vi "Digital_Write_3_Lines_2011.vi"() -> ()   [LabVIEW 2011]
uses:
  <vilib>/DAQmx/write.llb/DAQmx Write (Digital Bool 1Line 1Point).vi
  <vilib>/DAQmx/create/channels.llb/DAQmx Create Channel (DO-Digital Output).vi
  <vilib>/DAQmx/miscellaneous.llb/DAQmx Fill In Error Info.vi
panel:
  in  "Stop":bool
  in  "Line 1 Data":bool
  in  "Line 2 Data":bool
  in  "Line 3 Data":bool
  in  "Output Line 3":tag="Dev1/port0/line2"
  in  "Output Line 2":tag="Dev1/port0/line1"
  in  "Output Line 1":tag="Dev1/port0/line0"
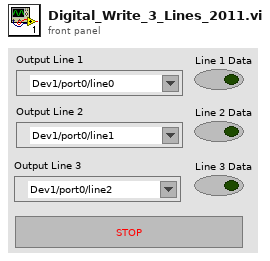
[diagram p1: front panel]
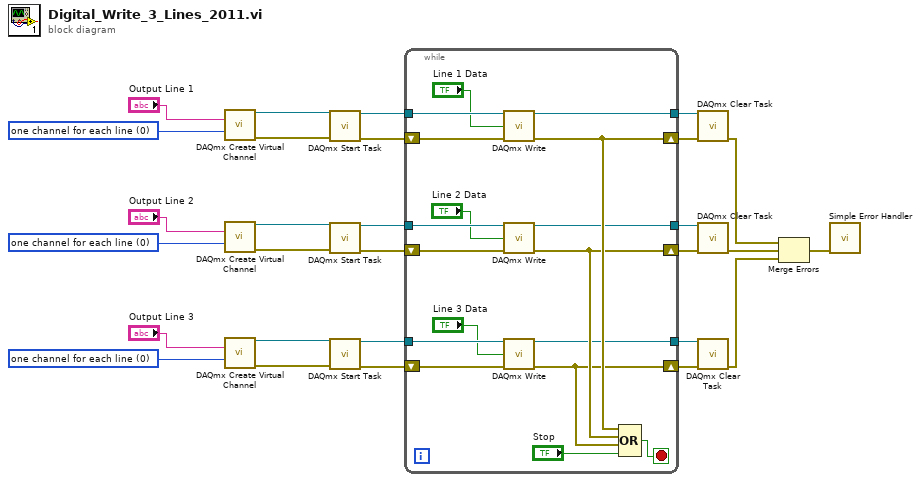
[diagram p0: block diagram]
diagram:
  w15 = 0 items=["one channel for each line", "one channel for all lines"] ("line grouping")
  w18 = 0 items=["one channel for each line", "one channel for all lines"] ("line grouping")
  w27 = 0 items=["one channel for each line", "one channel for all lines"] ("line grouping")
  n1 = call-poly <vilib>:"DAQmx Create Virtual Channel.vi"("lines"="Output Line 1", "line grouping"=w27) -> ("task out"=w26:refnum<k21>, "error out"=w25:errorcluster)  [unwired: 12 in]
  n2 = call-poly <vilib>:"DAQmx Create Virtual Channel.vi"("lines"="Output Line 2", "line grouping"=w18) -> ("task out"=w19:refnum<k21>, "error out"=w20:errorcluster)  [unwired: 12 in]
  n3 = call-poly <vilib>:"DAQmx Create Virtual Channel.vi"("lines"="Output Line 3", "line grouping"=w15) -> ("task out"=w14:refnum<k21>, "error out"=w13:errorcluster)  [unwired: 12 in]
  n4 = call <vilib>:"DAQmx Start Task.vi"("task/channels in"=w26, "error in"=w25) -> ("task out"=w24:refnum<k21>, "error out"=w23:errorcluster)  [unwired: 12 in]
  n5 = call <vilib>:"DAQmx Start Task.vi"("task/channels in"=w19, "error in"=w20) -> ("task out"=w21:refnum<k21>, "error out"=w22:errorcluster)  [unwired: 12 in]
  n6 = call <vilib>:"DAQmx Start Task.vi"("task/channels in"=w14, "error in"=w13) -> ("task out"=w12:refnum<k21>, "error out"=w11:errorcluster)  [unwired: 12 in]
  n7 = while {
    tunnel: w24 -> [w45]
    tunnel: w21 -> [w42]
    tunnel: w12 -> [w41]
    tunnel: [w31] -> w10
    tunnel: [w30] -> w8
    tunnel: [w29] -> w6
    shift-right: [w34] -> w7
    shift-left: w22 -> [w43]
    shift-right: [w35] -> w9
    shift-left: w23 -> [w44]
    shift-right: [w33] -> w5
    shift-left: w11 -> [w40]
    stop <- w36 stop-if-true
    n8 = call-poly <vilib>:"DAQmx Write.vi"("task/channels in"=w45, "data"="Line 1 Data", "error in"=w44) -> ("task out"=w31:refnum<k21>, "error out"=w35:errorcluster)  [unwired: 10 in, 1 out]
    n9 = call-poly <vilib>:"DAQmx Write.vi"("task/channels in"=w42, "data"="Line 2 Data", "error in"=w43) -> ("task out"=w30:refnum<k21>, "error out"=w34:errorcluster)  [unwired: 10 in, 1 out]
    n10 = call-poly <vilib>:"DAQmx Write.vi"("task/channels in"=w41, "data"="Line 3 Data", "error in"=w40) -> ("task out"=w29:refnum<k21>, "error out"=w33:errorcluster)  [unwired: 10 in, 1 out]
    n11 = Compound Arithmetic op=OR(w35, w34, w33, "Stop") -> (w36:bool)
  }
  n12 = call <vilib>:"DAQmx Clear Task.vi"("task in"=w10, "error in"=w9) -> ("error out"=w3:errorcluster)  [unwired: 13 in]
  n13 = call <vilib>:"DAQmx Clear Task.vi"("task in"=w8, "error in"=w7) -> ("error out"=w4:errorcluster)  [unwired: 13 in]
  n14 = call <vilib>:"DAQmx Clear Task.vi"("task in"=w6, "error in"=w5) -> ("error out"=w2:errorcluster)  [unwired: 13 in]
  n15 = Merge Errors(w3, w4, w2) -> (w1:errorcluster)
  n16 = call <vilib>:"Simple Error Handler.vi"("error in (no error)"=w1) -> ()  [unwired: 4 in, 5 out]
